vi "lectura de potenciometro con linxs.vi"() -> ()   [LabVIEW 2016]
uses:
  <vilib>/MakerHub/LINX/Public/Peripherals/Analog/Analog Read 1 Chan.vi
  <vilib>/MakerHub/LINX/Public/Peripherals/Digital/Digital Write 1 Chan.vi
  <vilib>/MakerHub/LINX/Public/Peripherals/Analog/Analog Read N Chans.vi
  <vilib>/MakerHub/LINX/Public/Peripherals/Digital/Digital Write N Chans.vi
  <vilib>/MakerHub/LINX/Private/Local IO/LinxAnalogRead.vi
  <vilib>/MakerHub/LINX/Public/Utilities/Check Channel.vi
  <vilib>/MakerHub/LINX/Private/Local IO/LinxDigitalWrite.vi
  <vilib>/MakerHub/LINX/Public/Utilities/Open Serial.vi
  <vilib>/MakerHub/LINX/Private/Utilties/Generate Error.vi
  <vilib>/MakerHub/LINX/LMH-LINX.lvlib
panel:
  in  "stop":bool
  out "Led":bool
  out "Meter":dbl(knob) scale=0.0..5.0
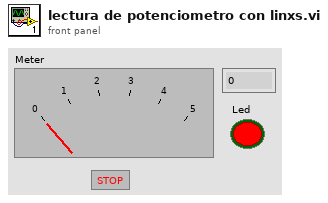
[diagram p1: front panel]
types:
  T1 = typedef "LMH-LINX.lvlib/LINX Ref.ctl" = cluster{"IO":T2, "Interface":T3, "LINX Device Config":T4}
  T2 = typedef "LMH-LINX.lvlib/Platform.ctl" = enum16{"Remote", "Local"}
  T3 = typedef "LMH-LINX.lvlib/Interface.ctl" = enum16{"Serial", "TCP"}
  T4 = typedef "LMH-LINX.lvlib/Device.lvlib/LINX Device Config.ctl" = cluster{"Interface":T3, "COM Port":refnum<visa-resource-name>, "TCP Configuration":T5, "Device Family":u8, "Device ID":u8, "Device Name":string, "TCP Ref":refnum<k5>, "Channels":T6}
  T5 = typedef "LMH-LINX.lvlib/Device.lvlib/TCP Config.ctl" = cluster{"IP Address":string, "Port":u16}
  T6 = typedef "LMH-LINX.lvlib/Channels.ctl" = cluster{"DI":u8[], "DO":u8[], "AI":u8[], "AO":u8[], "PWM":u8[], "QE":u8[], "UART":u8[], "I2C 2":u8[], "SPI":u8[], "CAN":u8[], "Servo":u8[], "AI Ref (V)":dbl, "AI Resolution (Bits)":u8, "AO Ref (V)":dbl, "AO Resolution (Bits)":u8}
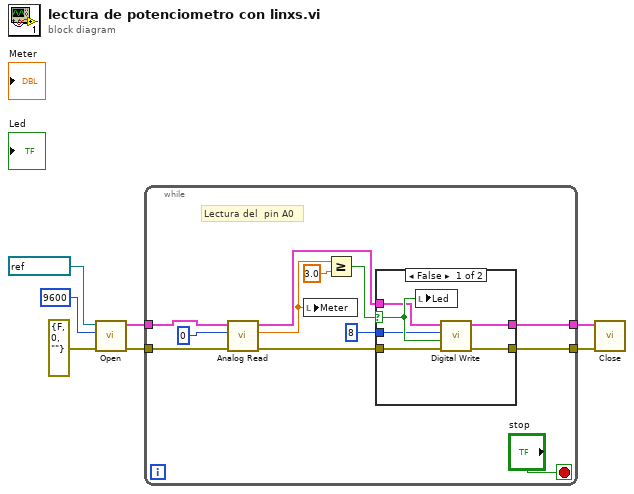
[diagram p0: block diagram]
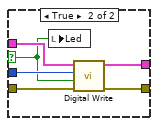
[diagram p2: hidden frame]
diagram:
  n1 = call-poly <vilib>:"Open.vi"("Error In"=errorcluster {"status"=FALSE, "code"=0, "source"=""}, "Baud Rate Override"=u32 9600, "Serial Port"=refnum<visa-resource-name> "COM6") -> ("Error Out"=w3:errorcluster, "LINX Resource"=w4:T1)  [unwired: 6 in, 1 out]
  n2 = while {
    tunnel: w4 -> [w18]
    tunnel: w3 -> [w17]
    tunnel: [w9] -> w2
    tunnel: [w8] -> w1
    stop <- "stop" stop-if-true
    # "Lectura del  pin A0"
    n3 = call-poly <vilib>:"Analog Read.vi"("Error In"=w17, "Analog Channel"=u8 0, "LINX Resource"=w18) -> ("Error Out"=w11:errorcluster, "Voltage"=w15:dbl, "LINX Resource"=w12:T1)  [unwired: 5 in, 1 out]
    n4 = local write "Meter"(w15) -> ()
    n5 = Greater Or Equal?(x=w15, y=3.0) -> (x >= y?=w13:bool)
    n6 = case shown="False" w13 {
      selector: w13 -> [w23 w28]
      tunnel: w12 -> [w21 w31]
      tunnel: w11 -> [w22 w30]
      tunnel: u8 8 ("DO Channel") -> [w20 w29]
      tunnel: [w25 w27] -> w9
      tunnel: [w24 w26] -> w8
      frame False {
        n7 = local write "Led"(w23) -> ()
        n8 = call-poly <vilib>:"Digital Write.vi"("Error In"=w22, "Output Value"=w23, "DO Channel"=w20, "LINX Resource"=w21) -> ("Error Out"=w24:errorcluster, "LINX Resource"=w25:T1)  [unwired: 6 in]
      }
      frame True {
        n9 = local write "Led"(w28) -> ()
        n10 = call-poly <vilib>:"Digital Write.vi"("Error In"=w30, "Output Value"=w28, "DO Channel"=w29, "LINX Resource"=w31) -> ("Error Out"=w26:errorcluster, "LINX Resource"=w27:T1)  [unwired: 6 in]
      }
    }
  }
  n11 = call <vilib>:"Close.vi"("Error In"=w1, "LINX Resource"=w2) -> ()  [unwired: 9 in, 1 out]
